vi "MotionProfile.vi"() -> ()   [LabVIEW 2016]
uses:
  Autonomous VIs/Autonomous Commands/Autonomous Support VIs/MotionProfile TypeDef.ctl
panel:
  in  "Total Points in File":dbl
  in  "Path Name":string
  out "Pre-Buffer Completed":bool
  in  "Motion Profile TypeDef":T1={"Left MP Array"=[[0.0, 0.0, 40.0], [-0.077273, -0.001545, 40.0], [-0.108484, -0.005885, 40.0], [-0.18078, -0.013116, 40.0], [-0.253035, -0.023237, 40.0], [-0.325234, -0.036247, 40.0], [-0.39736, -0.052141, 40.0], [-0.469397, -0.070917, 40.0], [-0.54133, -0.09257, 40.0], [-0.613144, -0.117096, 40.0], [-0.684824, -0.144489, 40.0], [-0.756356, -0.174743, 40.0], [-0.827727, -0.207852, 40.0], [-0.898925, -0.243809, 40.0], [-0.969942, -0.282607, 40.0], [-1.04077, -0.324238, 40.0], [-1.111405, -0.368694, 40.0], [-1.181847, -0.415968, 40.0], [-1.252101, -0.466052, 40.0], [-1.322176, -0.518939, 40.0], [-1.392092, -0.574623, 40.0], [-1.461872, -0.633097, 40.0], [-1.531551, -0.69436, 40.0], [-1.565612, -0.756984, 40.0], [-1.56423, -0.819553, 40.0], [-1.563056, -0.882075, 40.0], [-1.5621, -0.944559, 40.0], [-1.561375, -1.007014, 40.0], [-1.560887, -1.06945, 40.0], [-1.560644, -1.131876, 40.0], [-1.560648, -1.194302, 40.0], [-1.560899, -1.256738, 40.0], [-1.561396, -1.319193, 40.0], [-1.562134, -1.381679, 40.0], [-1.563106, -1.444203, 40.0], [-1.564301, -1.506775, 40.0], [-1.565708, -1.569403, 40.0], [-1.567314, -1.632096, 40.0], [-1.569103, -1.69486, 40.0], [-1.571061, -1.757703, 40.0], [-1.573168, -1.820629, 40.0], [-1.57541, -1.883646, 40.0], [-1.577767, -1.946756, 40.0], [-1.580223, -2.009965, 40.0], [-1.58276, -2.073276, 40.0], [-1.585364, -2.13669, 40.0], [-1.588018, -2.200211, 40.0], [-1.590707, -2.263839, 40.0], [-1.593419, -2.327576, 40.0], [-1.596141, -2.391422, 40.0], [-1.598861, -2.455376, 40.0], [-1.568244, -2.518106, 40.0], [-1.500958, -2.578144, 40.0], [-1.43021, -2.635353, 40.0], [-1.359116, -2.689717, 40.0], [-1.287697, -2.741225, 40.0], [-1.215973, -2.789864, 40.0], [-1.143968, -2.835623, 40.0], [-1.071701, -2.878491, 40.0], [-0.999195, -2.918459, 40.0], [-0.926471, -2.955517, 40.0], [-0.853548, -2.989659, 40.0], [-0.780446, -3.020877, 40.0], [-0.707182, -3.049164, 40.0], [-0.633776, -3.074515, 40.0], [-0.560244, -3.096925, 40.0], [-0.486602, -3.116389, 40.0], [-0.412867, -3.132904, 40.0], [-0.339052, -3.146466, 40.0], [-0.265174, -3.157073, 40.0], [-0.191246, -3.164723, 40.0], [-0.117283, -3.169414, 40.0], [-0.043298, -3.171146, 40.0], [-0.003151, -3.171272, 40.0], [0.0, -3.171272, 40.0]], "Left MP Index"=0.0, "Semaphore"=FALSE, "Right MP Array"=[[0.0, 0.0, 40.0], [-0.077273, -0.001545, 40.0], [-0.123334, -0.006479, 40.0], [-0.205584, -0.014702, 40.0], [-0.287874, -0.026217, 40.0], [-0.37022, -0.041026, 40.0], [-0.45264, -0.059131, 40.0], [-0.535147, -0.080537, 40.0], [-0.617759, -0.105248, 40.0], [-0.700489, -0.133267, 40.0], [-0.783354, -0.164601, 40.0], [-0.866366, -0.199256, 40.0], [-0.949539, -0.237238, 40.0], [-1.032883, -0.278553, 40.0], [-1.116409, -0.323209, 40.0], [-1.200123, -0.371214, 40.0], [-1.284029, -0.422575, 40.0], [-1.368127, -0.4773, 40.0], [-1.452413, -0.535397, 40.0], [-1.536876, -0.596872, 40.0], [-1.621499, -0.661732, 40.0], [-1.706255, -0.729982, 40.0], [-1.791111, -0.801627, 40.0], [-1.834317, -0.874999, 40.0], [-1.835697, -0.948427, 40.0], [-1.836871, -1.021902, 40.0], [-1.837825, -1.095415, 40.0], [-1.83855, -1.168957, 40.0], [-1.839037, -1.242518, 40.0], [-1.83928, -1.31609, 40.0], [-1.839276, -1.389661, 40.0], [-1.839025, -1.463222, 40.0], [-1.838528, -1.536763, 40.0], [-1.837791, -1.610274, 40.0], [-1.836821, -1.683747, 40.0], [-1.835627, -1.757172, 40.0], [-1.834221, -1.830541, 40.0], [-1.832617, -1.903846, 40.0], [-1.830829, -1.977079, 40.0], [-1.828874, -2.050234, 40.0], [-1.826768, -2.123305, 40.0], [-1.824529, -2.196286, 40.0], [-1.822174, -2.269173, 40.0], [-1.819721, -2.341962, 40.0], [-1.817185, -2.414649, 40.0], [-1.814584, -2.487233, 40.0], [-1.811933, -2.55971, 40.0], [-1.809246, -2.63208, 40.0], [-1.806536, -2.704341, 40.0], [-1.803817, -2.776494, 40.0], [-1.801098, -2.848538, 40.0], [-1.761028, -2.918979, 40.0], [-1.680356, -2.986193, 40.0], [-1.596564, -3.050056, 40.0], [-1.513117, -3.11058, 40.0], [-1.429995, -3.16778, 40.0], [-1.347176, -3.221667, 40.0], [-1.264639, -3.272253, 40.0], [-1.182362, -3.319547, 40.0], [-1.100324, -3.36356, 40.0], [-1.018504, -3.4043, 40.0], [-0.936883, -3.441776, 40.0], [-0.855441, -3.475993, 40.0], [-0.774159, -3.50696, 40.0], [-0.69302, -3.53468, 40.0], [-0.612008, -3.559161, 40.0], [-0.531104, -3.580405, 40.0], [-0.450295, -3.598417, 40.0], [-0.369564, -3.613199, 40.0], [-0.288897, -3.624755, 40.0], [-0.208279, -3.633086, 40.0], [-0.127697, -3.638194, 40.0], [-0.047136, -3.64008, 40.0], [-0.00343, -3.640217, 40.0], [0.0, -3.640217, 40.0]], "Right MP Index"=0.0}
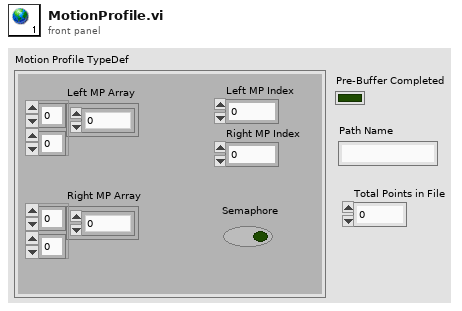
[diagram p1: front panel]
types:
  T1 = typedef "MotionProfile TypeDef.ctl" = cluster{"Left MP Array":dbl[][], "Left MP Index":dbl, "Semaphore":bool, "Right MP Array":dbl[][], "Right MP Index":dbl}
diagram:
